vi "Add Message-Subaddress Pair.vi"(4 "create timestamp channel":bool, 5 "message type":T2="BC to RT", 6 "parameters":T4(array[cluster]), 7 "number of words":u16=1, 8 "error in":errorcluster, 9 "remote terminal":T5, 10 "name":string, 11 "port":T1 format="%.0x") -> (0 "error out":errorcluster, 1 "message":T1=18446744073709551615 format="%.0x", 2 "subaddress":T1=18446744073709551615 format="%.0x", 3 "port out":T1 format="%.0x")   [LabVIEW 2020, in "AIM MIL-STD-1553 Scripting.lvlib"]
doc: "Adds an <b>subaddress</b> to the <b>remote terminal</b>, and a matching <b>message</b> to the Bus Controller within the <b>port</b>, including <b>parameters</b>, <b>number of words</b>, and the <b>create timestamp channel</b> setting in each. Determines the direction based on the <b>message type</b> (BC to RT/RT to BC). \n\nIt is recommended to call wrappers of this VI, <b>Add Message-Subaddress Pair (BC to RT).vi</b>, or <b>Add Message-Subaddress Pair (RT to BC).vi</b>, instead of this VI."
uses:
  AIM MIL-STD-1553 Scripting.lvlib
  <vilib>/NI VeriStand/Custom Device API/Custom Device Item Ref.ctl
  Shared/Terminal Endpoint.ctl
  Shared/Address.ctl
  Shared/Parameter Definition.ctl
  Shared/Message Type.ctl
  Shared/Direction.ctl
  <vilib>/NI VeriStand/Custom Device API/Custom Device API.lvlib
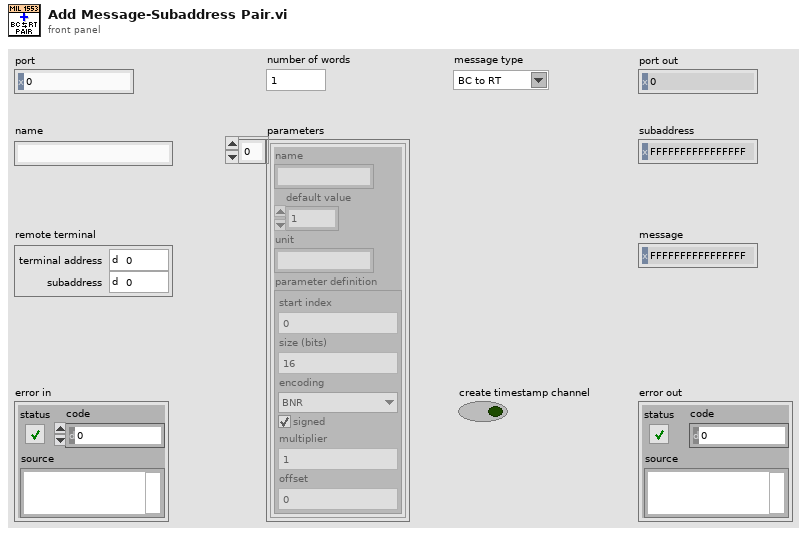
[diagram p1: front panel]
types:
  T1 = typedef "Custom Device API.lvlib/Custom Device Item Ref.ctl" = u64
  T2 = typedef "Message Type.ctl" = string
  T3 = typedef "Parameter Definition.ctl" = cluster{"start index":i32, "size (bits)":i32, "encoding":enum16{"BNR", "BCD", "Discrete"}, "signed":bool, "multiplier":dbl, "offset":dbl}
  T4 = cluster{"name":string, "default value":dbl, "unit":string, "parameter definition":T3}[]
  T5 = typedef "Terminal Endpoint.ctl" = cluster{"terminal address":T6, "subaddress":T6}
  T6 = typedef "Address.ctl" = u16
  T7 = typedef "Direction.ctl" = enum16{"Rx", "Tx"}
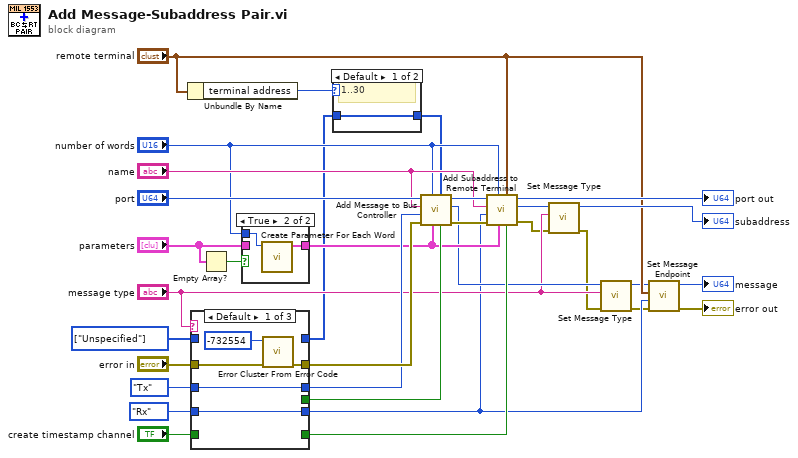
[diagram p0: block diagram]
diagram:
  w10 = enum16{"Rx", "Tx", "Unspecified"}[] [enum."Unspecified"] items=["Rx", "Tx", "Unspecified"] ("status channels directions")
  n1 = Unbundle By Name("remote terminal") -> ("terminal address"=w9:T6)
  n2 = case shown="Default" "message type" {
    tunnel: "error in" -> [w37 w43 w46]
    tunnel: Direction."Tx" -> [w35 w42 w48]
    tunnel: Direction."Rx" ("direction") -> [w34 w41 w47]
    tunnel: [w35 w41 w48] -> w22
    tunnel: [w34 w42 w47] -> w4
    tunnel: [w36 w43 w46] -> w26
    tunnel: [_ _ w45] -> w18
    tunnel: [_ w40 _] -> w24
    tunnel: "create timestamp channel" -> [_ w40 w45]
    tunnel: [_ w39 w44] -> w7
    tunnel: w10 -> [_ w39 w44]
    frame Default {
      n3 = call <vilib>:"Error Cluster From Error Code.vi"("error in (no error)"=w37, "error code (0)"=-732554) -> ("error out"=w36:errorcluster)  [unwired: 7 in]
    }
    frame "RT to BC" {
    }
    frame "BC to RT" {
    }
  }
  n4 = Empty Array?(array="parameters") -> (empty?=w31:bool)
  n5 = case shown="True" w31 {
    tunnel: "number of words" -> [_ w51]
    tunnel: "parameters" -> [w49 _]
    tunnel: [w49 w50] -> w19
    frame False {
    }
    frame True {
      n6 = call "Create Parameter For Each Word.vi"("number of words"=w51) -> ("parameters"=w50:T4)  [unwired: 9 in, 1 out]
    }
  }
  n7 = case shown="Default" w9 {
    tunnel: [w52 _] -> w8
    tunnel: w7 -> [w52 _]
    frame Default {
      # "1..30"
    }
    frame 31 {
      # "Broadcast"
    }
  }
  n8 = call "Add Message to Bus Controller.vi"("create timestamp channel"=w24, "status channels directions"=w8, "parameters"=w19, "number of words"="number of words", "error in"=w26, "direction"=w22, "name"="name", "port"="port") -> ("error out"=w33:errorcluster, "message"=w14:T1, "port out"=w21:T1)  [unwired: 1 in]
  n9 = call "Add Subaddress to Remote Terminal.vi"("create timestamp channel"=w18, "remote terminal"="remote terminal", "parameters"=w19, "number of words"="number of words", "error in"=w33, "direction"=w4, "name"="name", "port"=w21) -> ("error out"=w12:errorcluster, "subaddress"=w16:T1, "port out"=→"port out":T1)  [unwired: 1 in]
  n10 = call "Set Message Type.vi"("error in"=w12, "message type"="message type", "message or subaddress"=w16) -> ("error out"=w11:errorcluster, "message or subaddress out"=→"subaddress":T1)  [unwired: 7 in]
  n11 = call "Set Message Type.vi"("error in"=w11, "message type"="message type", "message or subaddress"=w14) -> ("error out"=w1:errorcluster, "message or subaddress out"=w3:T1)  [unwired: 7 in]
  n12 = call "Set Message Endpoint.vi"("error in"=w1, "direction"=w4, "remote terminal endpoint"="remote terminal", "message"=w3) -> ("error out"=→"error out":errorcluster, "message out"=→"message":T1)  [unwired: 6 in]
